vi "Write RAW File.vi"(5 "nA per B":i32, 6 "Brtn_extra/2":dbl, 7 "nAT per B":i32, 8 "error constant":errorcluster, 10 "Data In":u16[][](array[numeric]), 11 "refnum in":refnum<file>) -> (0 "error out":errorcluster, 3 "refnum out":refnum<file>)   [LabVIEW 2017]
panel:
  out "subarray":u16[](graph)
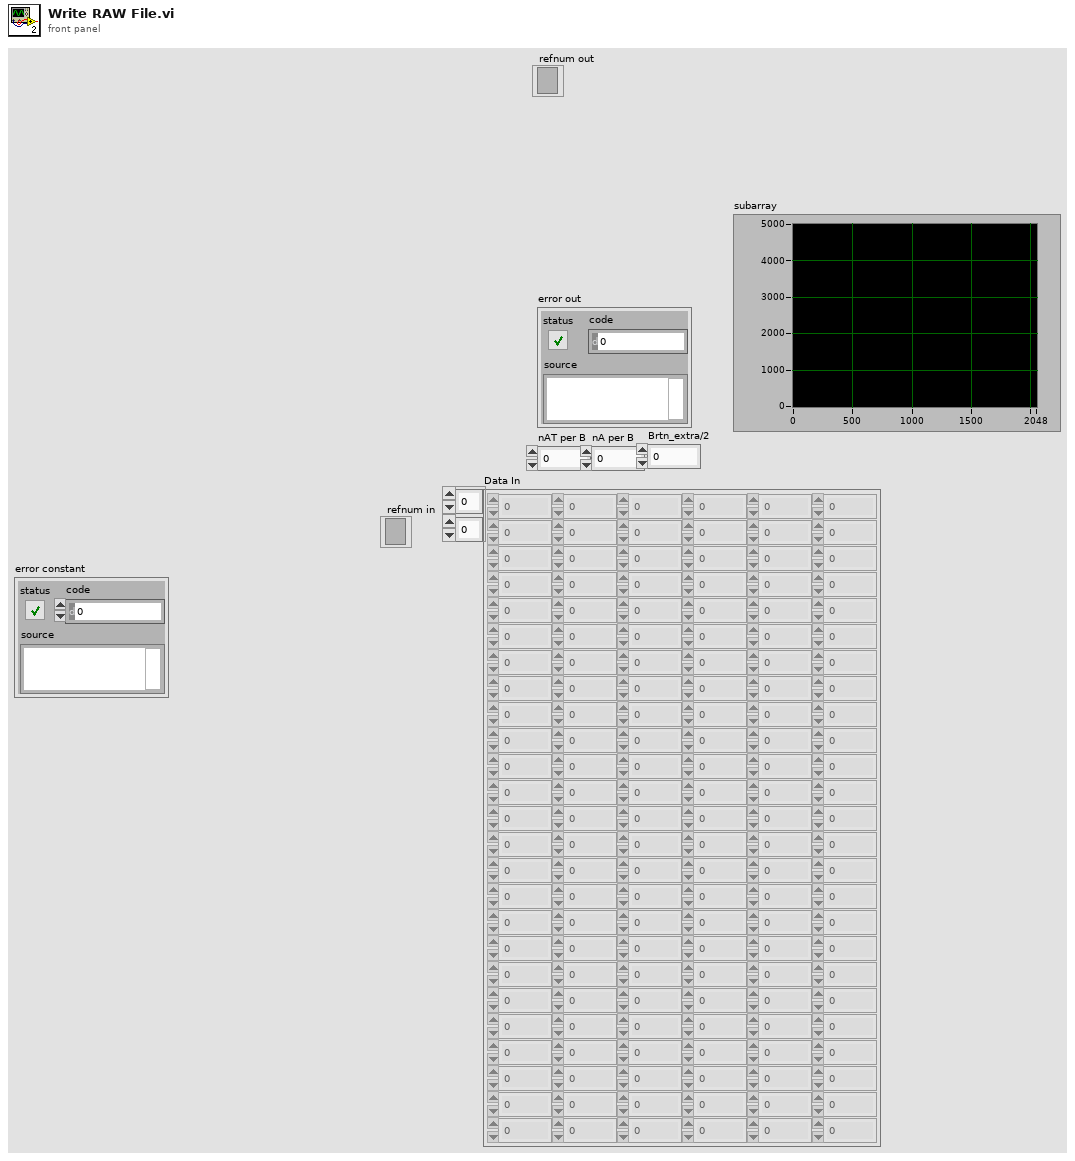
[diagram p1: front panel]
types:
  T1 = enum16{"big-endian, network order", "native, host order", "little-endian"}
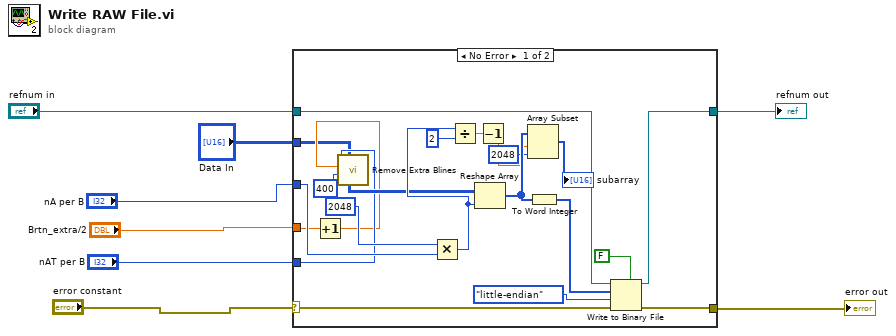
[diagram p0: block diagram]
diagram:
  n1 = case shown="No Error" "error constant" {
    selector: "error constant" -> [w29 w31]
    tunnel: "refnum in" -> [w26 w32]
    tunnel: [w28 w32] -> w3
    tunnel: [w30 w31] -> w4
    tunnel: "nA per B" -> [w22 _]
    tunnel: "Brtn_extra/2" -> [w10 _]
    tunnel: "nAT per B" -> [w12 _]
    tunnel: "Data In" -> [w9 _]
    frame No Error {
      n2 = Increment(x=w10) -> (x+1=w11:dbl)
      n3 = call "Remove Extra Blines.vi"("Data In"=w9, "#Aline"=400, "Start index"=w11, "nAT per B"=w12) -> ("Data Out"=w14:u16[][])  [unwired: 6 in]
      n4 = Multiply(x=2048 ("dimension size"), y=w22) -> (x*y=w18:i32)
      n5 = Divide(x=w18, y=2) -> (x/y=w16:dbl)
      n6 = Reshape Array(w14, w18) -> (w21:u16[])
      n7 = Decrement(x=w16) -> (x-1=w15:dbl)
      n8 = Array Subset(array=w21, index=w15, length=2048) -> (→"subarray":u16[])
      n9 = To Word Integer(number=w21) -> (16bit integer=w24:i16[])
      n10 = Write to Binary File(file (use dialog)=w26, data=w24, error in=w29, 5:FALSE ("prepend array or string size? (T)"), 9:T1."little-endian" ("byte order (0:big-endian, network order)")) -> (refnum out=w28:refnum<file>, error out=w30:errorcluster)  [unwired: 1 in, 1 out]
    }
    frame Error {
    }
  }
  "error out" <- w4
  "refnum out" <- w3
